vi "ObtainQueue.vi"(6 "ModuleNumber":i32, 8 "错误输入（无错误）":errorcluster, 10 "ModuleName":string) -> (0 "错误输出":errorcluster, 3 "MessageQueue":refnum<queue>)   [LabVIEW 2019, in "module.lvlib"]
uses:
  module.lvlib
  Message.ctl
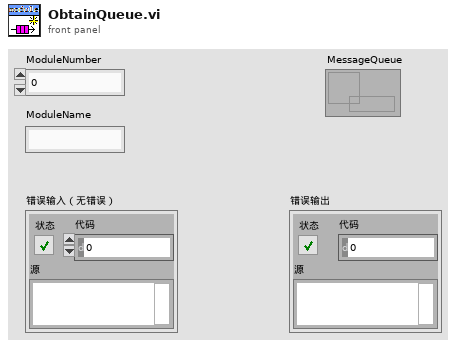
[diagram p1: front panel]
types:
  T1 = typedef "module.lvlib/Message.ctl" = cluster{"Message":string, "Message Data":variant}
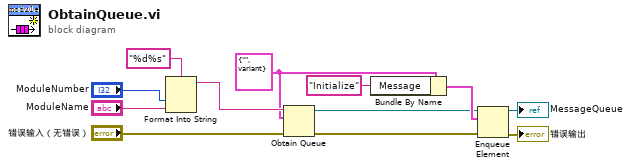
[diagram p0: block diagram]
diagram:
  w6 = T1 {"Message"="", "Message Data"=variant} ("Message")
  n1 = Format Into String(format string="%d%s" ("格式字符串"), "ModuleNumber", "ModuleName") -> (resulting string=w9:string)  [unwired: 2 in, 1 out]
  n2 = Obtain Queue(name (unnamed)=w9, element data type=w6, error in (no error)="错误输入（无错误）") -> (queue out=w4:refnum<queue>, error out=w7:errorcluster)  [unwired: 2 in, 1 out]
  n3 = Bundle By Name(cluster=w6, "Message"="Initialize") -> (w5:T1)
  n4 = Enqueue Element(queue=w4, element=w5, error in (no error)=w7) -> (queue out=→"MessageQueue":refnum<queue>, error out=→"错误输出":errorcluster)  [unwired: 1 in, 1 out]
